vi "Calculate DNL.vi"(9 "1 Ideal LSB value":dbl, 11 "DAC Analog readings":dbl[](array[numeric]) format="%#.8p") -> (1 "DNL index":i32, 2 "DNL":dbl, 3 "DNL waveform":dbl[](graph))   [LabVIEW 2021, in "Linearity_DAC.lvlib"]
uses:
  Linearity_DAC.lvlib
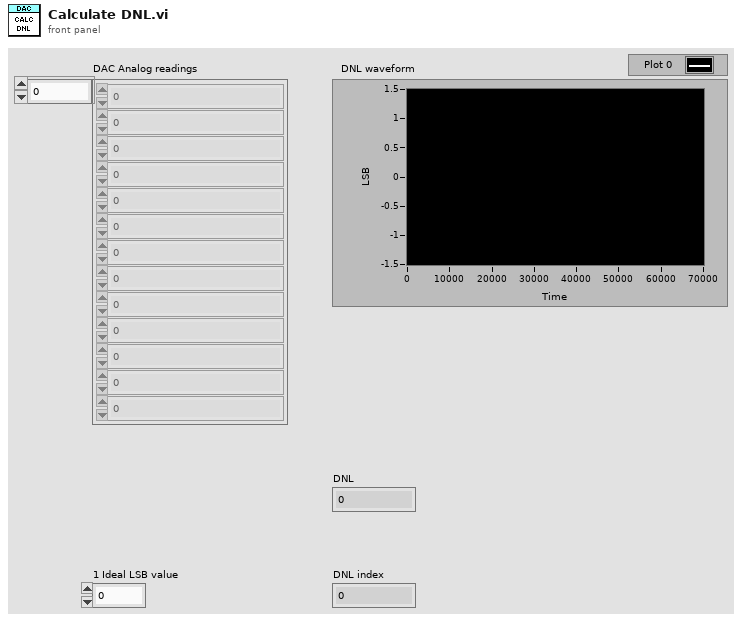
[diagram p1: front panel]
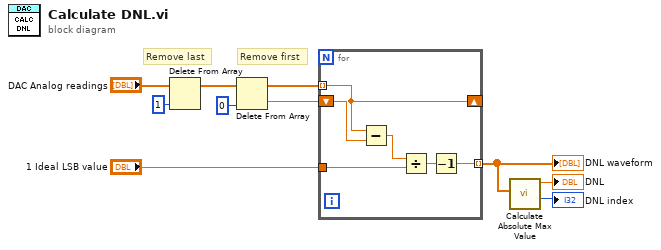
[diagram p0: block diagram]
diagram:
  # "Remove last"
  # "Remove first"
  n1 = Delete From Array(array="DAC Analog readings", length=1) -> (array with subset deleted=w6:dbl[])  [unwired: 1 in, 1 out]
  n2 = Delete From Array(array=w6, index=0) -> (deleted portion=w3:dbl, array with subset deleted=w9:dbl[])  [unwired: 1 in]
  n3 = for {
    tunnel: w9 -> [w15] mode=indexing
    shift-right: [w15] -> _
    shift-left: w3 -> [w16]
    tunnel: [w12] -> w4 mode=indexing
    tunnel: "1 Ideal LSB value" -> [w11]
    n4 = Subtract(x=w15, y=w16) -> (x-y=w13:dbl)
    n5 = Divide(x=w13, y=w11) -> (x/y=w14:dbl)
    n6 = Decrement(x=w14) -> (x-1=w12:dbl)
  }
  "DNL waveform" <- w4
  n7 = call "Calculate Absolute Max Value.vi"("Data"=w4) -> ("Abs max index"=→"DNL index":i32, "Abs max value"=→"DNL":dbl)  [unwired: 9 in]
